vi "dataProcess_wavelengthMeter.vi"(0 "reference":refnum<class "OSA.lvclass">, 1 "Interferogram":sgl[](array[numeric]) format="%.2f", 2 "x min":sgl format="%.2f", 3 "x max":sgl format="%.2f", 4 "length":u32, 5 "error in (no error)":errorcluster) -> (14 "duplicate reference":refnum<class "OSA.lvclass">, 19 "error out":errorcluster)   [LabVIEW 2010, in "OSA.lvclass"]
doc: "Calculates wavelength by interferogram cycle-counting. See also dataAcq_get_wavelengthMeter.vi, (FTSLib.dll: FTS_GetLastWavelengthmeter_Wavenr)."
uses:
  OSA.lvclass
  OSA20X_misc.lvlib
  FTSLib.dll
panel:
  in  "waveNr  dummy":sgl
  out "waveNr  (/cm)":sgl format="%.2f"
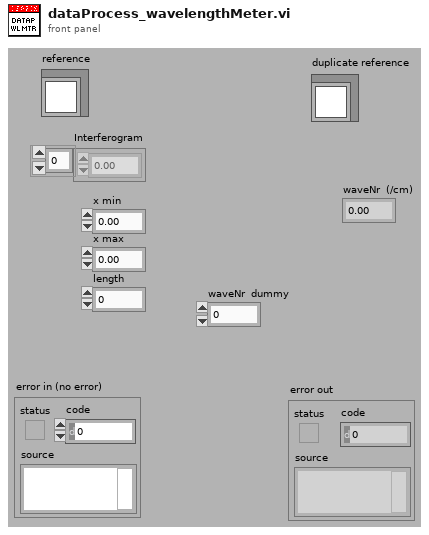
[diagram p1: front panel]
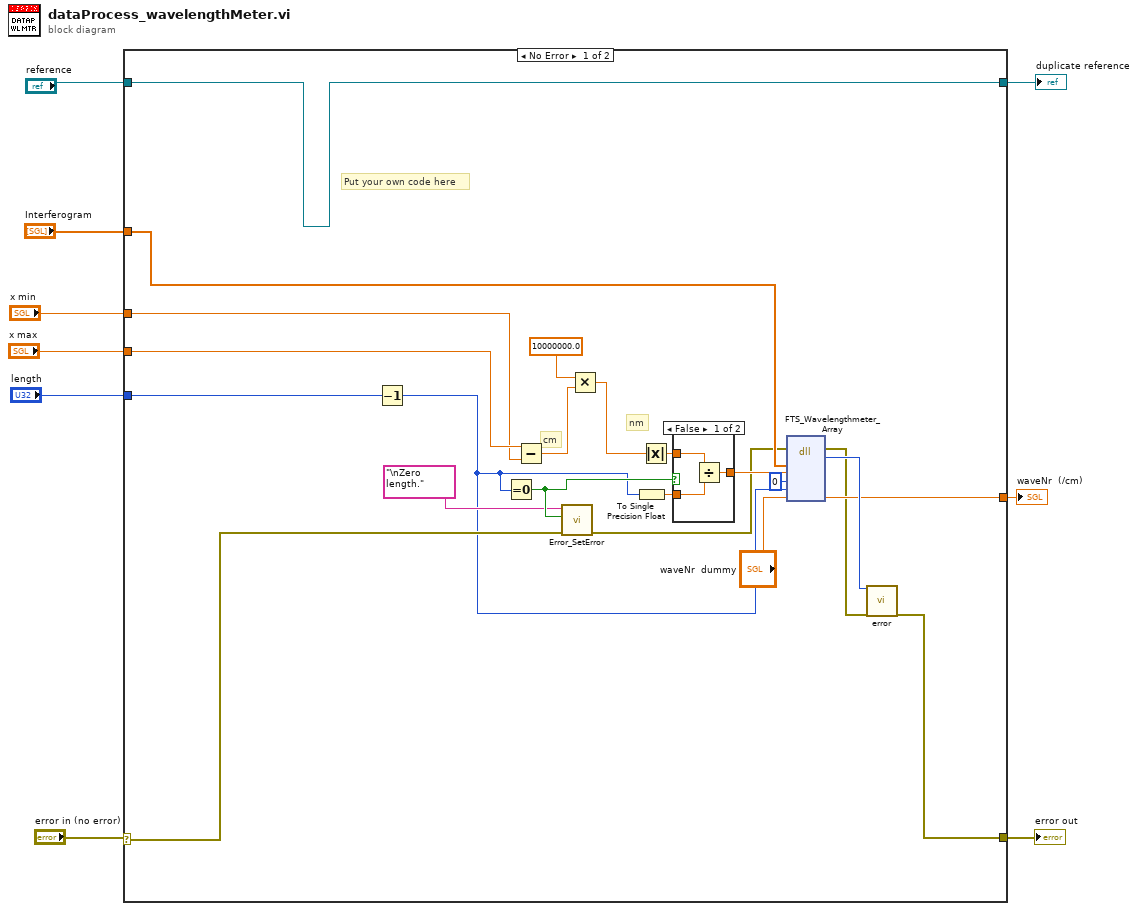
[diagram p0: block diagram]
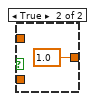
[diagram p2: hidden frame]
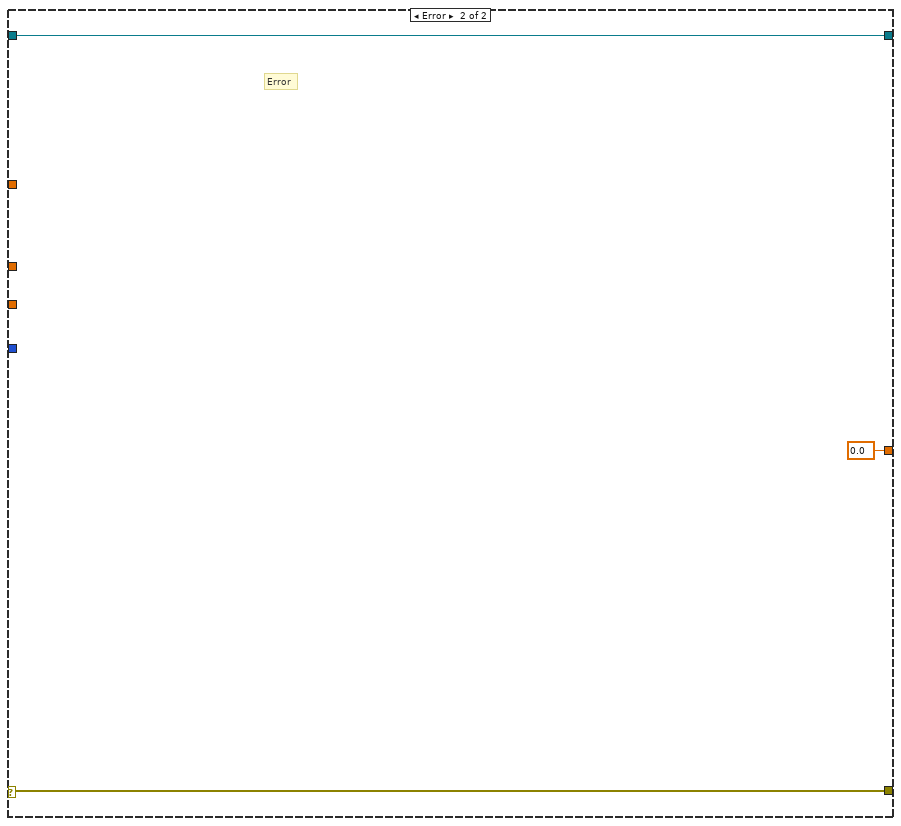
[diagram p3: hidden frame]
diagram:
  n1 = case shown="No Error" "error in (no error)" {
    selector: "error in (no error)" -> [w21 w37]
    tunnel: [w30 w37] -> w9
    tunnel: "reference" -> [w24 w38]
    tunnel: [w24 w38] -> w6
    tunnel: "Interferogram" -> [w29 _]
    tunnel: "x min" -> [w22 _]
    tunnel: "x max" -> [w23 _]
    tunnel: "length" -> [w20 _]
    tunnel: [w13 sgl 0.0 ("waveNr")] -> w1
    frame No Error {
      # "nm"
      # "cm"
      # "Put your own code here"
      n2 = Decrement(x=w20) -> (x-1=w14:u32)
      n3 = Equal To 0?(x=w14) -> (x = 0?=w28:bool)
      n4 = Subtract(x=w23, y=w22) -> (x-y=w17:sgl)
      n5 = call "Error_SetError.vi"("error in"=w21, "status (true)"=w28, "source(\"\")"="\nZero length." ("source(\"\")")) -> ("error out"=w11:errorcluster)  [unwired: 4 in]
      n6 = Multiply(x=sgl 10000000.0, y=w17) -> (x*y=w18:sgl)
      n7 = To Single Precision Float(number=w14) -> (single precision float=w27:sgl)
      n8 = Absolute Value(x=w18) -> (abs(x)=w25:sgl)
      n9 = case shown="False" w28 {
        tunnel: w25 -> [w34 _]
        tunnel: w27 -> [w33 _]
        tunnel: [w32 sgl 1.0] -> w16
        frame False {
          n10 = Divide(x=w34, y=w33) -> (x/y=w32:sgl)
        }
        frame True {
        }
      }
      n11 = dll-call lib="FTSLib.dll" fn="FTS_Wavelengthmeter_Array"(error in=w11, "interferogramData"=w29, "sampleDistance"=w16, "startIdx"=u32 0, "stopIdx"=w14, "waveNr"="waveNr  dummy") -> (error out=w10:errorcluster, "return type"=w31:i32, "waveNr"=w13:sgl)  [unwired: 6 in, 1 out]
      n12 = call "error.vi"("result code"=w31, "error in (no error)"=w10) -> ("error out"=w30:errorcluster)  [unwired: 15 in, 2 out]
    }
    frame Error {
      # "Error"
    }
  }
  "error out" <- w9
  "duplicate reference" <- w6
  "waveNr  (/cm)" <- w1
